vi "Word_Insert_Link.vi"(0 "Word._Document":refnum<k7>, 1 "Address":string, 2 "Subaddress":string, 3 "font":T1 {"font size" format="%.2f"; "strike through" items=["Strk Unchanged", "Strk Yes", "Strk No"]; "underline" items=["Und Unchanged", "Und Yes", "Und No"]; "italic" items=["Ital Unchanged", "Ital Yes", "Ital No"]; "bold" items=["Bold Unchanged", "Bold Yes", "Bold No"]}, 5 "Text to display":string, 7 "Start":i32, 9 "End":i32, 11 "Error in":errorcluster, 12 "Insertion point":u16(ring)=1 items=["begining of document", "end of document", "bookmark", "Custom"], 13 "bookmark name":string) -> (8 "Start out":i32, 10 "End out":i32, 15 "Error out":errorcluster)   [LabVIEW 2020, in "NI_ReportGenerationToolkit.lvlib"]
uses:
  <vilib>/addons/_office/NI_ReportGenerationToolkit.lvlib
  <vilib>/addons/_office/_exclsub.llb/font.ctl
panel:
  # "Position"
  # "Content"
  # "Output"
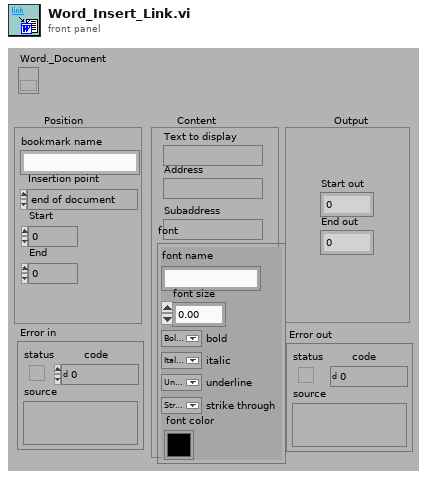
[diagram p1: front panel]
types:
  T1 = typedef "NI_ReportGenerationToolkit.lvlib/font.ctl" = cluster{"font name":string, "font size":dbl, "bold":u16, "italic":u16, "underline":u16, "strike through":u16, "font color":u32}
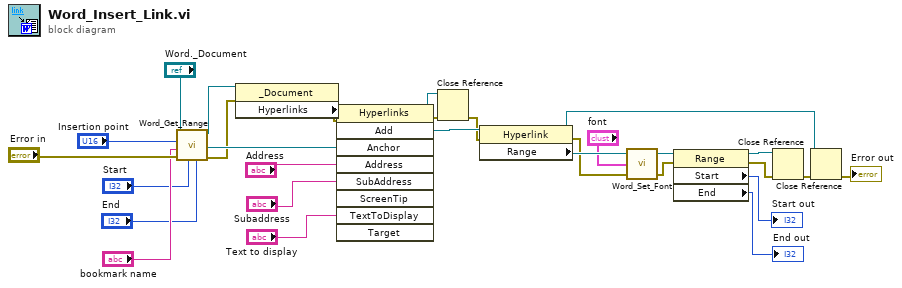
[diagram p0: block diagram]
diagram:
  n1 = call <vilib>:"Word_Get_Range.vi"("end"="End", "start"="Start", "error in"="Error in", "bookmark name"="bookmark name", "insertion point"="Insertion point", "document in"="Word._Document") -> ("error out (no error)"=w21:errorcluster, "range"=w22:refnum<k7>, "document out"=w25:refnum<k7>)  [unwired: 3 out]
  n2 = property class="_Document"(reference=w25, error in=w21) -> (error out=w28:errorcluster, "Hyperlinks"=w27:refnum<k7>)  [unwired: 1 out]
  n3 = invoke class="Hyperlinks" method="Add"(reference=w27, error in=w28, "Anchor"=w22, "Address"="Address", "SubAddress"="Subaddress", "TextToDisplay"="Text to display") -> (reference out=w13:refnum<k7>, error out=w15:errorcluster, "Add"=w23:refnum<k7>)  [unwired: 3 in, 6 out]
  n4 = Close Reference(reference=w13, error in (no error)=w15) -> (error out=w14:errorcluster)
  n5 = property class="Hyperlink"(reference=w23, error in=w14) -> (reference out=w16:refnum<k7>, error out=w19:errorcluster, "Range"=w20:refnum<k7>)
  n6 = call <vilib>:"Word_Set_Font.vi"("Range in"=w20, "font"="font", "Error in"=w19) -> ("Range out"=w8:refnum<k7>, "Error out"=w7:errorcluster)  [unwired: 5 out]
  n7 = property class="Range"(reference=w8, error in=w7) -> (reference out=w6:refnum<k7>, error out=w5:errorcluster, "Start"=→"Start out":i32, "End"=→"End out":i32)
  n8 = Close Reference(reference=w6, error in (no error)=w5) -> (error out=w18:errorcluster)
  n9 = Close Reference(reference=w16, error in (no error)=w18) -> (error out=→"Error out":errorcluster)
